vi "prefPageGlobals.vi"() -> ()   [LabVIEW 2016]
panel:
  in  "default tag prefix":string="getDefault->"
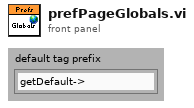
[diagram p1: front panel]
diagram:
